vi "Util_LibraryGlobals.vi"() -> ()   [LabVIEW 2019, in "Trajectory_Library.lvlib"]
doc: "THIS IS AN INTERNAL ROUTINE. DO NOT CALL OR USE DIRECTLY FROM USER CODE.\n\nThis stores global variables for this library. Currently it is used to store use counts for\ninformation reported to the Field Management System via the ReportUsage WPI call.\n\nNote: It only contains items that currently have IDs to be reported. Things like splines and \ntrajectories are currently not included in that list."
uses:
  Trajectory_Library.lvlib
panel:
  out "LibUsage_LinearFIlter":i32 format="%20.0f"
  out "LibUsage_PIDController":i32 format="%20.0f"
  out "LibUsage_ProfiledPID":i32 format="%20.0f"
  out "LibUsage_Kinematics":i32 format="%20.0f"
  out "LibUsage_Odometry":i32 format="%20.0f"
  out "LibUsage_TrapezoidProfile":i32 format="%20.0f"
  # "THIS IS AN INTERNAL ROUTINE.  DO NOT USE DIRECTLY OUTSIDE\nOF THE LIBRARY."
  # "There are the only items in the WPILIB usage reporting that match items\nin this library."
  # "Could add -- SlewRateFilter, MedianFilter, Ramsete, various Feedforward,\n                        Trajectory, Spline."
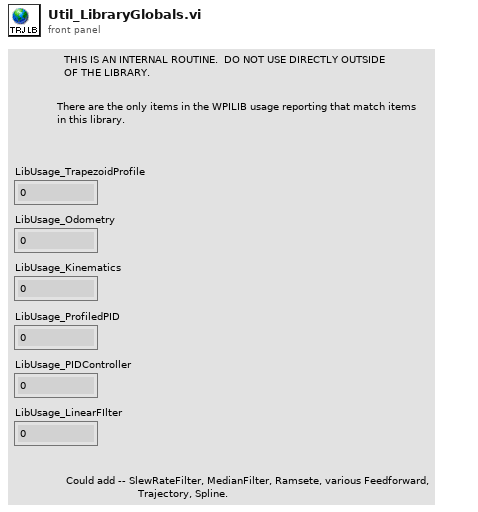
[diagram p1: front panel]
diagram:
